vi "EDIT DUE DATE.vi"(0 "DATA IN":T1[](array[typedef]), 1 "REFERENCES":T2) -> (7 "DATA OUT":T1[](array[typedef]))   [LabVIEW 2019]
uses:
  Controls/References Cluster.ctl
  <vilib>/userDefined/High Color/IMAQdx.ctl
  Controls/Custom Calendar/Custom Calendar.xctl
  Controls/Table Data Types/Inventory Data Type.ctl
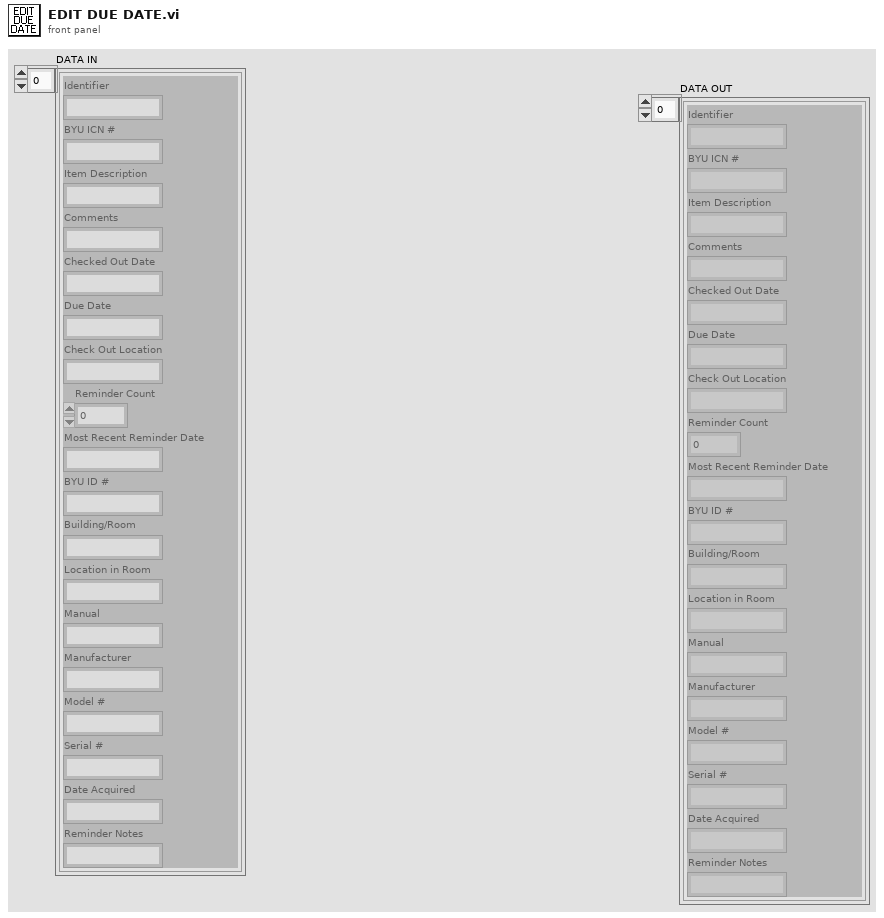
[diagram p1: front panel]
types:
  T1 = typedef "Inventory Data Type.ctl" = cluster{"Identifier":string, "BYU ICN #":string, "Item Description":string, "Comments":string, "Checked Out Date":string, "Due Date":string, "Check Out Location":string, "Reminder Count":i32, "Most Recent Reminder Date":string, "BYU ID #":string, "Building/Room":string, "Location in Room":string, "Manual":string, "Manufacturer":string, "Model #":string, "Serial #":string, "Date Acquired":string, "Reminder Notes":string}
  T2 = typedef "References Cluster.ctl" = cluster{"MAIN PAGES":refnum<vi>, "ADD/EDIT ITEM REFERENCES":cluster{"Identifier":refnum<vi>, "BYU ICN #":refnum<vi>, "Item Description":refnum<vi>, "Comments":refnum<vi>, "Checked Out Date":refnum<vi>, "Due Date":refnum<vi>, "Check Out Location":refnum<vi>, "Reminder Count":refnum<vi>, "Most Recent Reminder Date":refnum<vi>, "BYU ID #":refnum<vi>, "Building/Room":refnum<vi>, "Location in Room":refnum<vi>, "Manual":refnum<vi>, "Manufacturer":refnum<vi>, "Model #":refnum<vi>, "Serial #":refnum<vi>, "Date Acquired":refnum<vi>, "ADD/EDIT ITEM LABEL":refnum<vi>, "ARCHIVE ITEM":refnum<vi>, "Archive Item Inputs":refnum<vi>, "Reminder Notes":refnum<vi>}, "ADD/EDIT USER REFERENCES":cluster{"BYU ID # (##-###-####)":refnum<vi>, "First Name":refnum<vi>, "Last Name":refnum<vi>, "Phone Number (###-###-####)":refnum<vi>, "Email":refnum<vi>, "Department":refnum<vi>, "Graduation Status":refnum<vi>, "Anticipated Graduation Year":refnum<vi>, "Credit Score":refnum<vi>, "Date Added":refnum<vi>, "Graduation Clearance Date":refnum<vi>, "Picture File Name":refnum<vi>, "ADD/EDIT USER LABEL":refnum<vi>, "Department Map":refnum<vi>, "Status Map":refnum<vi>, "Anticipated Graduation Year Map":refnum<vi>, "User Agreement":refnum<vi>, "User Comments":refnum<vi>, "Camera":refnum<vi>}, "RETURN ITEM REFERENCES":cluster{"Item or Person:":refnum<vi>, "Search Return Results":refnum<vi>, "What are you searching for?":refnum<vi>}, "SEARCH DATABASE REFERENCES":cluster{"What to Search For:":refnum<vi>, "Where to Search":refnum<vi>, "Column to Search In":refnum<vi>, "Column to Sort By":refnum<vi>, "Search Database Results":refnum<vi>, "Inventory Column Selector":refnum<vi>, "User Column Selector":refnum<vi>, "Inventory Archive Column Selector":refnum<vi>, "User Archive Column Selector":refnum<vi>, "Sales Tracking Column Selector":refnum<vi>, "Checked In Archive Column Selector":refnum<vi>, "Restore User":refnum<vi>, "Date Range":refnum<vi>, "Dates Less Than":refnum<vi>, "Dates Greater Than":refnum<vi>, "Search Print Receipt":refnum<vi>}, "USER ITEMS REFERENCES":cluster{"USER'S INFORMATION":refnum<vi>, "User's Checked Out Items":refnum<vi>, "User Info Comments":refnum<vi>, "SEE USER INFO COMMENTS":refnum<vi>}, "EDIT ITEMS REFERENCES":cluster{"New Check Out Location":refnum<vi>, "Items to Edit":refnum<vi>, "Edit Items Due Date":refnum<vi>, "New Reminder Notes":refnum<vi>, "New Item Description":refnum<vi>}, "CHECK OUT ITEMS REFERENCES":cluster{"Enter Item:":refnum<vi>, "Check Out Items Due Date":refnum<vi>, "Check Out Location":refnum<vi>, "Items to be Checked Out":refnum<vi>, "Possible Items":refnum<vi>}, "TRANSFER ITEMS REFERENCES":cluster{"Search Parameter":refnum<vi>, "What to Match":refnum<vi>, "Matching Individuals":refnum<vi>, "Items to be Transferred":refnum<vi>}, "SETTINGS REFERENCES":cluster{"PSC Database Settings":refnum<vi>, "PSC Sales Item Spreadsheet":refnum<vi>}, "PSC SALES REFERENCES":cluster{"BYU ID CARD #":refnum<vi>, "Sale Description":refnum<vi>, "Scan or Enter Item Name":refnum<vi>, "Items to be Sold":refnum<vi>, "Grand Total":refnum<vi>, "Item List":refnum<vi>}}
  T3 = cluster{"Enter Item:":refnum<vi>, "Check Out Items Due Date":refnum<vi>, "Check Out Location":refnum<vi>, "Items to be Checked Out":refnum<vi>, "Possible Items":refnum<vi>}
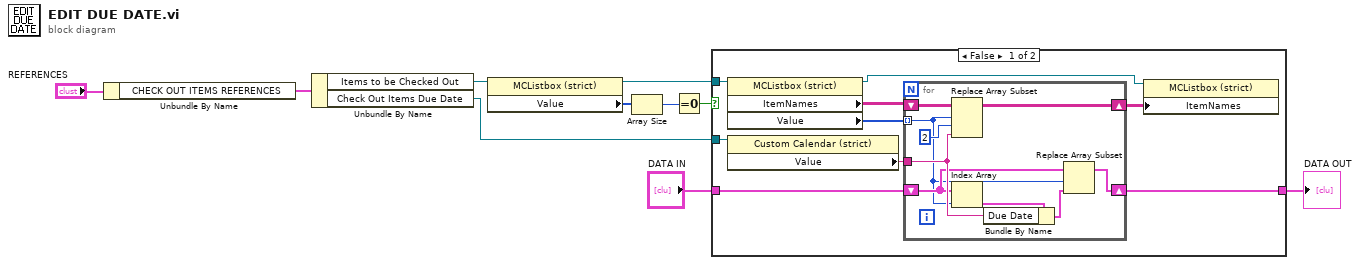
[diagram p0: block diagram]
diagram:
  n1 = Unbundle By Name("REFERENCES") -> ("CHECK OUT ITEMS REFERENCES"=w9:T3)
  n2 = Unbundle By Name(w9) -> ("Items to be Checked Out"=w8:refnum<vi>, "Check Out Items Due Date"=w3:refnum<vi>)
  n3 = property class="MCListbox (strict)"(reference=w8) -> (reference out=w4:refnum<vi>, "Value"=w7:i32[])  [unwired: 1 in, 1 out]
  n4 = Array Size(array=w7) -> (size(s)=w6:i32)
  n5 = Equal To 0?(x=w6) -> (x = 0?=w5:bool)
  n6 = case shown="False" w5 {
    tunnel: w4 -> [w19 _]
    tunnel: w3 -> [w16 _]
    tunnel: "DATA IN" -> [w12 w29]
    tunnel: [w11 w29] -> w1
    frame False {
      n7 = property class="MCListbox (strict)"(reference=w19) -> (reference out=w13:refnum<vi>, "ItemNames"=w18:string[][], "Value"=w17:i32[])  [unwired: 1 in, 1 out]
      n8 = property class="Custom Calendar (strict)"(reference=w16) -> ("Value"=w15:string)  [unwired: 1 in, 2 out]
      n9 = for {
        shift-right: [w26] -> w14
        shift-left: w18 -> [w28]
        tunnel: w17 -> [w22] mode=indexing
        tunnel: w15 -> [w24]
        shift-right: [w20] -> w11
        shift-left: w12 -> [w23]
        n10 = Replace Array Subset(array=w28, new element=w24, index (row)=w22, index (col)=2 ("disabled index (col)")) -> (w26:string[][])
        n11 = Index Array(array=w23, index=w22) -> (element=w25:T1)
        n12 = Bundle By Name(cluster=w25, "Due Date"=w24) -> (w21:T1)
        n13 = Replace Array Subset(array=w23, new element=w21, index=w22) -> (w20:T1[])
      }
      n14 = property class="MCListbox (strict)"(reference=w13, "ItemNames"=w14) -> ()  [unwired: 1 in, 2 out]
    }
    frame True {
    }
  }
  "DATA OUT" <- w1
